vi "SP Perform Filter Ripple Limit Testing.vi"(0 "Filter Limit":T12={"Limit #"=1, "Parameter"={"Stimulus Port"=1, "Response Port"=2}, "Format"=enum."Lin Mag", "Filter Type"=enum."Bandpass", "Passband"={"Start/Center"=510.0, "Stop/Span"=610.0, "Units"=enum."MHz", "Freq Format"=enum."Start/Stop", "Bandwidth Attn"=3.0, "Passband Limit"=FALSE}, "Ripple"={"Ripple Limit"=TRUE, "Window On"=TRUE, "Ripple"=0.1, "Window"=10.0, "Units"=enum."MHz"}, "Attenuation Points"=[], "Skirt Points"=[]} {"Parameter"."Stimulus Port" min=1 step=1; "Parameter"."Response Port" min=1 step=1; "Passband"."Bandwidth Attn" format="%.3g"; "Passband"."Stop/Span" format="%.3g"; "Passband"."Start/Center" format="%.3g"}, 5 "Data":T11={"F0"=500.0, "dF"=1.0, "Formatted Values"=[-6.0, -6.0, -6.0, -6.0, -6.0, -6.0, -5.0, -4.0, -3.0, -2.0, -1.0017226002993769, -0.8636286738753696, -1.012432061728755, -0.8135188671805874, -1.084383696215112, -1.192695586219516, -0.8228939725524264, -1.1588169801015764, -1.0069715761898415, -0.8118111488159718, -0.9516999033989667, -1.0842662636672022, -1.0261931083967077, -0.816874162233468, -0.8335770068326294, -1.1794529347576463, -1.1032959879886735, -1.197742447623333, -0.9631229100196212, -0.9908453124177325, -0.9835470980893588, -1.10217991844936, -0.8956607286257672, -0.8794782872077156, -0.9013683651609963, -1.0772188731817596, -0.992723355191172, -0.9536275499498994, -0.9874327685983141, -0.921963653527827, -0.8848787728556787, -1.1874980208218, -0.996957511881206, -0.9972503730309241, -0.8866139538542095, -1.07344181331393, -0.881559772443858, -1.0112449407130875, -0.9865384477979471, -0.9901446738263366, -1.1718630063784758, -0.9951725256878827, -0.931778781153855, -0.9846289731021831, -0.851763264124267, -0.9086965469391421, -0.8349429101974368, -0.8383742350256687, -1.106571816484691, -0.9554005266395742, -0.9376822403043366, -1.131287512516927, -1.0382288806403288, -0.917054052988136, -0.9489467877812984, -0.9264227759143271, -1.0918690925892351, -1.1668737446636852, -1.0021735712381068, -1.1541225361979714, -1.1931131329605709, -0.8730502330378824, -0.850411285659811, -1.137775166801135, -1.1870586525662095, -1.0926571181161528, -1.118993526927924, -1.1211410787283602, -0.8920697041785735, -0.888430731015914, -1.0656600076605476, -1.1666787859795846, -1.0713340188424678, -0.8625910088884297, -1.1434360227216422, -0.9217710376784376, -1.1218396445954617, -0.9558195687190933, -1.1773692443654946, -1.0827782751424972, -1.1567791336122029, -0.8684407402614696, -0.8177845157195978, -0.9040657051180614, -0.9313557288389804, -1.0236831450620423, -1.050426714979035, -0.8344777069605718, -0.8274082929927138, -1.1990080831766776, -1.0947798998491134, -1.1963114865246718, -1.0016247375583676, -1.0877110100652403, -1.1556028882288836, -1.1918380581525247, -0.9751292214691399, -0.8884133044813358, -1.0347444321214612, -0.9445125246491541, -2.0, -3.0, -4.0, -5.0, -6.0, -6.0, -6.0, -6.0, -6.0, -6.0]}, 9 "Generate Plot Output? (f)":bool, 11 "error in (no error)":errorcluster, 12 "Limit Results In":T2={"Limit #"=0, "Parameter"={"Stimulus Port"=1, "Response Port"=0}, "Bandwidth Pass?"={"Pass?"=FALSE, "Bandwidth"=0.0, "Limit"=0.0, "Units"=enum."Hz"}, "Ripple Pass?"={"Pass?"=FALSE, "Ripple"=0.0, "Limit"=0.0, "Format"=enum."Log Mag"}, "Attenuation Results"=[], "Skirt Results"=[], "Pass?"=FALSE} {"Parameter"."Stimulus Port" min=1 step=1; "Parameter"."Response Port" min=1 step=1}, 13 "Format":T1 caption="Display Format" items=["Log Mag", "Phase", "Expanded Phase", "Delay", "Smith", "Polar", "Lin Mag", "SWR", "Loss", "Real", "Imaginary"]) -> (1 "Upper Limits":cluster{"x values":dbl[], "y values":dbl[]}[](array[cluster]), 3 "Lower Limits":cluster{"x values":dbl[], "y values":dbl[]}[](array[cluster]), 4 "Limits Pass/Fail":cluster{"Upper Pass?":bool, "Lower Pass?":bool}, 6 "Upper and Lower Limits":T10, 10 "Failures":cluster{"x values":dbl[], "y values":dbl[]}[](array[cluster]), 14 "Limit Results Out":T2={"Limit #"=0, "Parameter"={"Stimulus Port"=1, "Response Port"=0}, "Bandwidth Pass?"={"Pass?"=FALSE, "Bandwidth"=0.0, "Limit"=0.0, "Units"=enum."Hz"}, "Ripple Pass?"={"Pass?"=FALSE, "Ripple"=0.0, "Limit"=0.0, "Format"=enum."Log Mag"}, "Attenuation Results"=[], "Skirt Results"=[], "Pass?"=FALSE} {"Parameter"."Stimulus Port" min=1 step=1; "Parameter"."Response Port" min=1 step=1}, 15 "error out":errorcluster)   [LabVIEW 2011]
uses:
  TypeDefs/SP Filter.ctl
  TypeDefs/SP Parameter.ctl
  TypeDefs/SP Format.ctl
  TypeDefs/SP Filter Type.ctl
  TypeDefs/SP Filter Passband.ctl
  TypeDefs/SP Frequency Units.ctl
  TypeDefs/SP Frequency Format.ctl
  TypeDefs/SP Filter Ripple.ctl
  TypeDefs/SP Attenuation Point.ctl
  TypeDefs/SP Attenuation Type.ctl
  TypeDefs/SP Skirt Rejection Point.ctl
  TypeDefs/SP Relative Loss.ctl
  TypeDefs/SP Limit Results.ctl
  TypeDefs/SP Bandwidth Limit Results.ctl
  TypeDefs/SP Ripple Limit Results.ctl
  TypeDefs/SP Attenuation Limit Results.ctl
  TypeDefs/SP Skirt Limit Results.ctl
  TypeDefs/SP Display Format.ctl
panel:
  out "Plot Output":cluster{"x values":dbl[], "y values":dbl[]}[](graph)
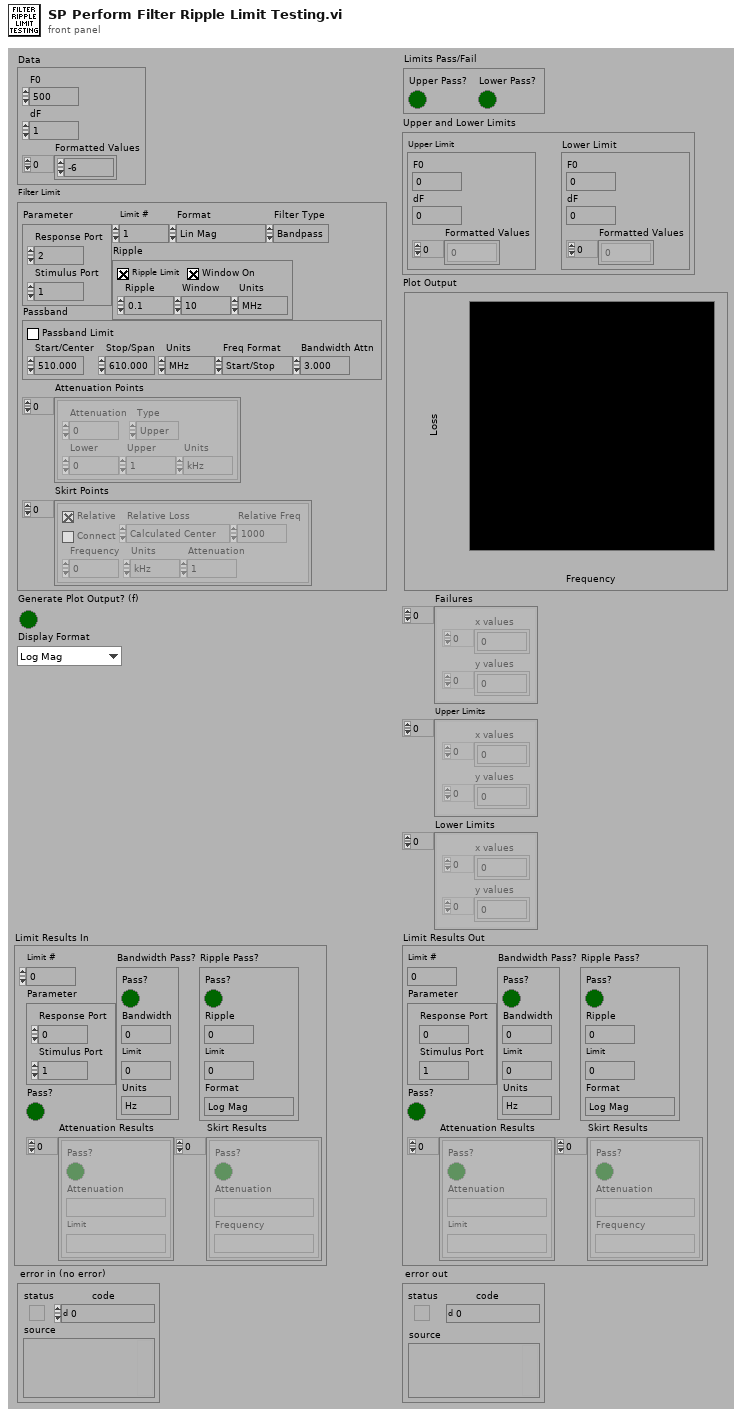
[diagram p1: front panel]
types:
  T1 = typedef "SP Display Format.ctl" = i32
  T2 = typedef "SP Limit Results.ctl" = cluster{"Limit #":i8, "Parameter":T3, "Bandwidth Pass?":T4, "Ripple Pass?":T6, "Attenuation Results":T8[], "Skirt Results":T9[], "Pass?":bool}
  T3 = typedef "SP Parameter.ctl" = cluster{"Stimulus Port":i8, "Response Port":i8}
  T4 = typedef "SP Bandwidth Limit Results.ctl" = cluster{"Pass?":bool, "Bandwidth":dbl, "Limit":dbl, "Units":T5}
  T5 = typedef "SP Frequency Units.ctl" = enum16{"Hz", "kHz", "MHz", "GHz", "Points"}
  T6 = typedef "SP Ripple Limit Results.ctl" = cluster{"Pass?":bool, "Ripple":dbl, "Limit":dbl, "Format":T7}
  T7 = typedef "SP Format.ctl" = enum16{"Log Mag", "Lin Mag", "SWR", "Phase", "Expanded Phase", "Delay", "Insertion Loss", "Isolation", "Return Loss"}
  T8 = typedef "SP Attenuation Limit Results.ctl" = cluster{"Pass?":bool, "Attenuation":string, "Limit":string}
  T9 = typedef "SP Skirt Limit Results.ctl" = cluster{"Pass?":bool, "Attenuation":string, "Frequency":string}
  T10 = cluster{"Upper Limit":cluster{"F0":dbl, "dF":dbl, "Formatted Values":dbl[]}, "Lower Limit":cluster{"F0":dbl, "dF":dbl, "Formatted Values":dbl[]}}
  T11 = cluster{"F0":dbl, "dF":dbl, "Formatted Values":dbl[]}
  T12 = typedef "SP Filter.ctl" = cluster{"Limit #":i8, "Parameter":T3, "Format":T7, "Filter Type":T13, "Passband":T14, "Ripple":T16, "Attenuation Points":T17[], "Skirt Points":T19[]}
  T13 = typedef "SP Filter Type.ctl" = enum16{"Lowpass", "Highpass", "Bandpass", "Bandstop"}
  T14 = typedef "SP Filter Passband.ctl" = cluster{"Start/Center":dbl, "Stop/Span":dbl, "Units":T5, "Freq Format":T15, "Bandwidth Attn":dbl, "Passband Limit":bool}
  T15 = typedef "SP Frequency Format.ctl" = enum16{"Start/Stop", "Center/Span"}
  T16 = typedef "SP Filter Ripple.ctl" = cluster{"Ripple Limit":bool, "Window On":bool, "Ripple":dbl, "Window":dbl, "Units":T5}
  T17 = typedef "SP Attenuation Point.ctl" = cluster{"Attenuation":dbl, "Type":T18, "Lower":dbl, "Upper":dbl, "Units":T5}
  T18 = typedef "SP Attenuation Type.ctl" = enum16{"Center", "Lower", "Upper"}
  T19 = typedef "SP Skirt Rejection Point.ctl" = cluster{"Relative":bool, "Connect":bool, "Frequency":dbl, "Units":T5, "Attenuation":dbl, "Relative Loss":T20, "Relative Freq":dbl}
  T20 = typedef "SP Relative Loss.ctl" = enum16{"Calculated Center", "Passband Minimum", "Passband Maximum", "Passband Average", "Frequency"}
  T21 = cluster{"x0":dbl, "dx":dbl, "Stored Values":dbl[]}
  T22 = cluster{cluster{"x0":dbl, "dx":dbl, "Stored Values":dbl[]}, cluster{"x0":dbl, "dx":dbl, "Stored Values":dbl[]}}
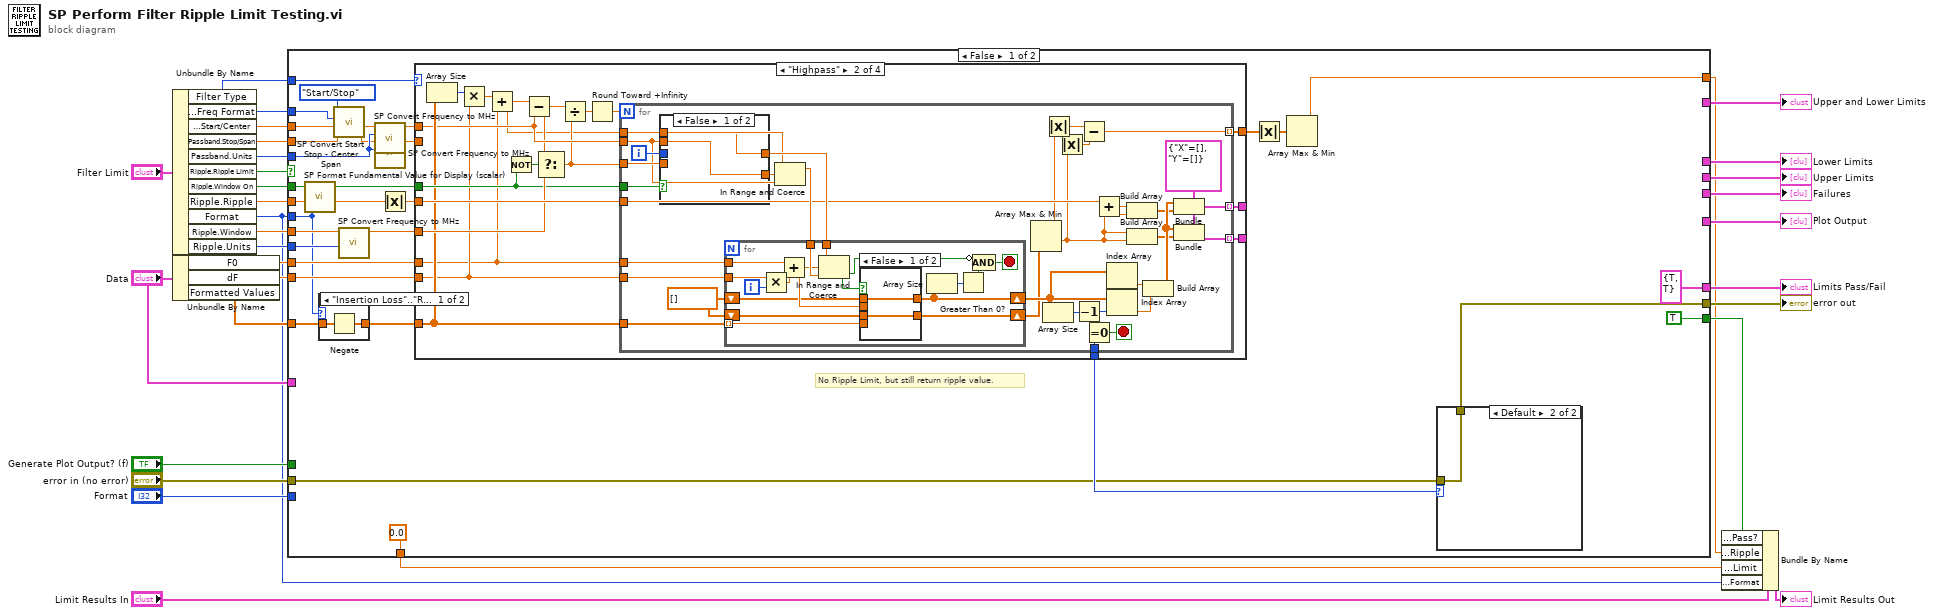
[diagram p0: block diagram]
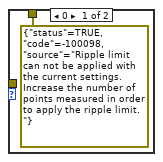
[diagram p3: hidden frame]
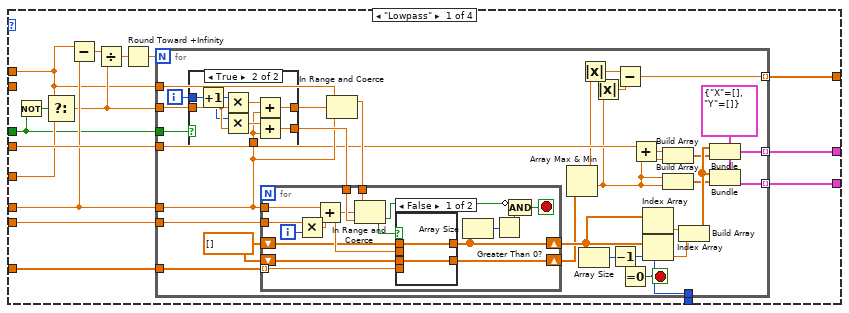
[diagram p4: hidden frame]
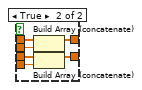
[diagram p6: hidden frame]
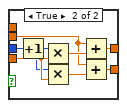
[diagram p7: hidden frame]
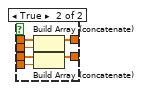
[diagram p8: hidden frame]
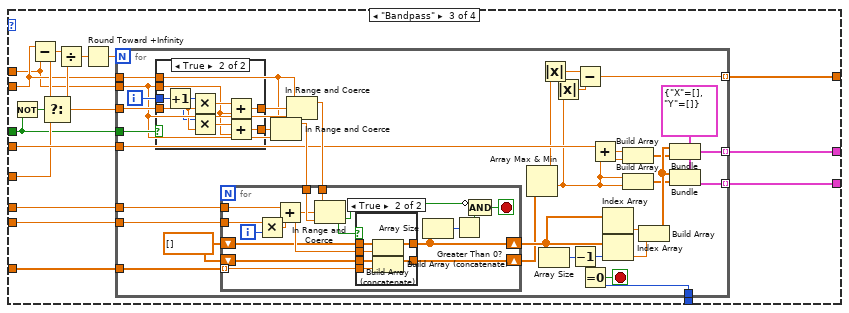
[diagram p9: hidden frame]
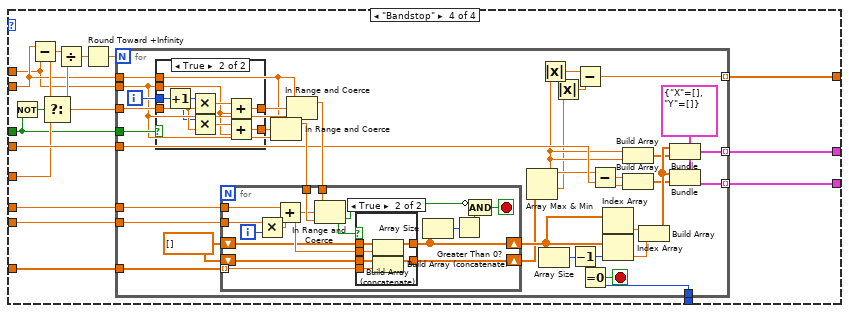
[diagram p12: hidden frame]
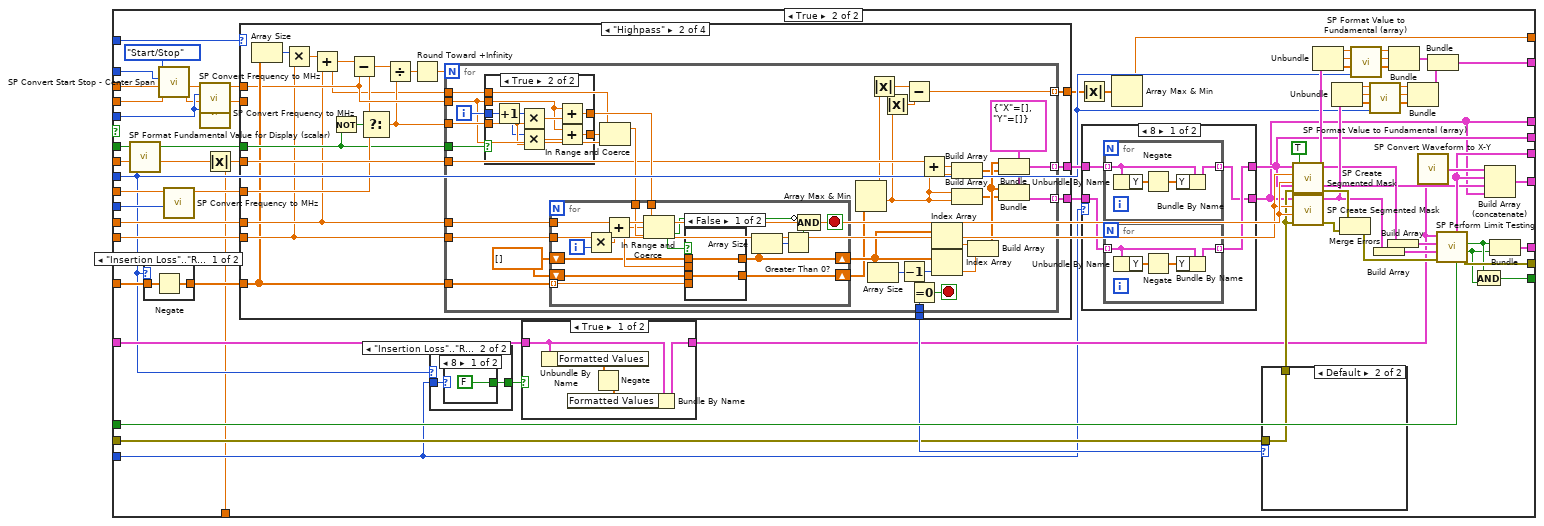
[diagram p15: hidden frame]
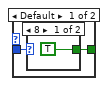
[diagram p17: hidden frame]
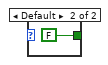
[diagram p18: hidden frame]
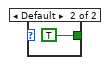
[diagram p19: hidden frame]
diagram:
  n1 = Unbundle By Name("Filter Limit") -> ("Filter Type"=w16:T13, "Passband.Freq Format"=w15:T15, "Passband.Start/Center"=w30:dbl, "Passband.Stop/Span"=w29:dbl, "Passband.Units"=w28:T5, "Ripple.Ripple Limit"=w25:bool, "Ripple.Window On"=w24:bool, "Ripple.Ripple"=w23:dbl, "Format"=w1:T7, "Ripple.Window"=w22:dbl, "Ripple.Units"=w21:T5)
  n2 = Unbundle By Name("Data") -> ("F0"=w27:dbl, "dF"=w26:dbl, "Formatted Values"=w20:dbl[])
  n3 = case shown="False" w25 {
    tunnel: w16 -> [w62 w465]
    tunnel: w30 -> [w52 w450]
    tunnel: w29 -> [w51 w449]
    tunnel: w28 -> [w61 w464]
    tunnel: w27 -> [w54 w452]
    tunnel: w26 -> [w53 w451]
    tunnel: w20 -> [w42 w418]
    tunnel: w24 -> [w55 w456]
    tunnel: w23 -> [w44 w420]
    tunnel: w22 -> [w58 w461]
    tunnel: w21 -> [w57 w460]
    tunnel: w1 -> [w40 w407]
    tunnel: "Data" -> [_ w409]
    tunnel: "Generate Plot Output? (f)" -> [_ w426]
    tunnel: [cluster{"Upper Pass?":bool, "Lower Pass?":bool} {"Upper Pass?"=TRUE, "Lower Pass?"=TRUE} w437] -> w9
    tunnel: [_ w442] -> w6
    tunnel: "error in (no error)" -> [w45 w424]
    tunnel: [w33 w458] -> w17
    tunnel: w15 -> [w47 w445]
    tunnel: [_ w412] -> w14
    tunnel: [_ w414] -> w13
    tunnel: [_ w440] -> w12
    tunnel: [TRUE w436] -> w4
    tunnel: [_ w427] -> w8
    tunnel: "Format" -> [_ w406]
    tunnel: [w37 w403] -> w3
    tunnel: [0.0 w402] -> w2
    frame False {
      # "No Ripple Limit, but still return ripple value."
      n4 = call "SP Format Fundamental Value for Display (scalar).vi"("Format"=w40, "Stored Value (0, linear)"=w44) -> ("Display Value"=w43:dbl)  [unwired: 5 out]
      n5 = case shown="\"Insertion Loss\"..\"Return Loss\"" w40 {
        tunnel: w42 -> [w64 w65]
        tunnel: [w63 w65] -> w41
        frame "Insertion Loss".."Return Loss" {
          n6 = Negate(x=w64) -> (-x=w63:dbl[])
        }
        frame Default {
        }
      }
      n7 = call "SP Convert Start Stop - Center Span.vi"("Stop/Span In"=w51, "Start/Center In"=w52, "Freq Format From"=w47, "Freq Format To"=SP_Frequency_Format."Start/Stop") -> ("Stop/Span Out"=w50:dbl, "Start/Center Out"=w49:dbl)  [unwired: 6 out]
      n8 = call "SP Convert Frequency to MHz.vi"("Units"=w57, "Frequency"=w58) -> ("Converted Frequency"=w56:dbl)  [unwired: 1 in, 8 out]
      n9 = call "SP Convert Frequency to MHz.vi"("Units"=w61, "Frequency"=w49) -> ("Converted Frequency"=w59:dbl)  [unwired: 1 in, 8 out]
      n10 = call "SP Convert Frequency to MHz.vi"("Units"=w61, "Frequency"=w50) -> ("Converted Frequency"=w60:dbl)  [unwired: 1 in, 8 out]
      n11 = Absolute Value(x=w43) -> (abs(x)=w36:dbl)
      n12 = case shown="\"Highpass\"" w62 {
        tunnel: w54 -> [w78 w153 w241 w325]
        tunnel: w53 -> [w82 w155 w242 w326]
        tunnel: w41 -> [w83 w159 w243 w327]
        tunnel: w60 -> [_ _ w238 w322]
        tunnel: w59 -> [w72 w158 w237 w321]
        tunnel: w56 -> [w79 w165 w248 w332]
        tunnel: [w71 w161 w245 w329] -> _
        tunnel: [w70 w160 w244 w328] -> _
        tunnel: w36 -> [w81 w167 w250 w334]
        tunnel: w55 -> [w73 w162 w246 w330]
        tunnel: [w69 w150 w235 w319] -> w46
        tunnel: [w68 w149 w234 w318] -> w38
        frame "Lowpass" {
          n13 = Not(x=w73) -> (.not. x?=w80:bool)
          n14 = Select(t=w72, s=w80, f=w79) -> (s? t:f=w76:dbl)
          n15 = Subtract(x=w72, y=w78) -> (x-y=w77:dbl)
          n16 = Divide(x=w77, y=w76) -> (x/y=w75:dbl)
          n17 = Round Toward +Infinity(x=w75) -> (ceil(x): smallest int >= x=w74:dbl)
          n18 = for {
            N: w74 -> [_]
            tunnel: w83 -> [w114]
            tunnel: [w106] -> w71 mode=indexing
            tunnel: [w105] -> w70 mode=indexing
            tunnel: w78 -> [w94]
            tunnel: w82 -> [w104]
            tunnel: w81 -> [w92]
            tunnel: w76 -> [w103]
            tunnel: w73 -> [w102]
            tunnel: w72 -> [w97]
            tunnel: [w89] -> w69
            tunnel: [w86] -> w68 mode=indexing
            i -> [w101]
            stop <- w90 stop-if-true
            w99 = dbl[] []
            w110 = cluster{"X":dbl[], "Y":dbl[]} {"X"=[], "Y"=[]} ("Cluster")
            n19 = case shown="True" w102 {
              tunnel: w94 -> [w116 w118]
              tunnel: [w115 w122] -> w96
              tunnel: w103 -> [w115 w121]
              tunnel: w101 -> [_ w120]
              tunnel: [w116 w117] -> w100
              frame False {
              }
              frame True {
                n20 = Increment(x=w120) -> (x+1=w124:i32)
                n21 = Multiply(x=w124, y=w121) -> (x*y=w123:dbl)
                n22 = Multiply(x=w120, y=w121) -> (x*y=w119:dbl)
                n23 = Add(x=w123, y=w118) -> (x+y=w122:dbl)
                n24 = Add(x=w119, y=w118) -> (x+y=w117:dbl)
              }
            }
            n25 = In Range and Coerce(upper limit=w97, x=w96, lower limit=w94) -> (coerced(x)=w95:dbl)  [unwired: 1 out]
            n26 = for {
              tunnel: w114 -> [w134] mode=indexing
              tunnel: w104 -> [w139]
              tunnel: w94 -> [w138]
              tunnel: w95 -> [w136]
              tunnel: w100 -> [w135]
              shift-right: [w132] -> w93
              shift-left: w99 -> [w133]
              shift-right: [w129] -> w98
              shift-left: w99 -> [w130]
              i -> [w140]
              stop <- w126 stop-if-true
              n27 = Multiply(x=w139, y=w140) -> (x*y=w137:dbl)
              n28 = Add(x=w138, y=w137) -> (x+y=w131:dbl)
              n29 = In Range and Coerce(upper limit=w136, x=w131, lower limit=w135) -> (In Range?=w127:bool)  [unwired: 1 out]
              n30 = case shown="False" w127 {
                tunnel: w134 -> [_ w148]
                tunnel: w133 -> [w142 w147]
                tunnel: [w142 w146] -> w132
                tunnel: w131 -> [_ w145]
                tunnel: w130 -> [w141 w144]
                tunnel: [w141 w143] -> w129
                frame False {
                }
                frame True {
                  n31 = Build Array (concatenate)(w144, w145) -> (w143:dbl[])
                  n32 = Build Array (concatenate)(w147, w148) -> (w146:dbl[])
                }
              }
              n33 = Array Size(array=w129) -> (size(s)=w128:i32)
              n34 = Greater Than 0?(x=w128) -> (x > 0?=w125:bool)
              n35 = Compound Arithmetic op=AND(invert w127, w125) -> (w126:bool)
            }
            n36 = Array Max & Min(array=w93) -> (max value=w84:dbl, min value=w85:dbl)  [unwired: 2 out]
            n37 = Array Size(array=w98) -> (size(s)=w113:i32)
            n38 = Absolute Value(x=w84) -> (abs(x)=w88:dbl)
            n39 = Absolute Value(x=w85) -> (abs(x)=w87:dbl)
            n40 = Decrement(x=w113) -> (x-1=w89:i32)
            n41 = Subtract(x=w88, y=w87) -> (x-y=w86:dbl)
            n42 = Equal To 0?(x=w89) -> (x = 0?=w90:bool)
            n43 = Add(x=w92, y=w85) -> (x+y=w91:dbl)
            n44 = Index Array(array=w98) -> (element=w112:dbl)  [unwired: 1 in]
            n45 = Index Array(array=w98, index=w89) -> (element=w111:dbl)
            n46 = Build Array(w91, w91) -> (w107:dbl[])
            n47 = Build Array(w85, w85) -> (w108:dbl[])
            n48 = Build Array(w112, w111) -> (w109:dbl[])
            n49 = Bundle(cluster=w110, "X"=w109, "Y"=w107) -> (w106:cluster{"X":dbl[], "Y":dbl[]})
            n50 = Bundle(cluster=w110, "X"=w109, "Y"=w108) -> (w105:cluster{"X":dbl[], "Y":dbl[]})
          }
        }
        frame "Highpass" {
          n51 = Array Size(array=w159) -> (size(s)=w156:i32)
          n52 = Multiply(x=w156, y=w155) -> (x*y=w154:dbl)
          n53 = Add(x=w154, y=w153) -> (x+y=w151:dbl)
          n54 = Not(x=w162) -> (.not. x?=w166:bool)
          n55 = Subtract(x=w151, y=w158) -> (x-y=w157:dbl)
          n56 = Select(t=w157, s=w166, f=w165) -> (s? t:f=w152:dbl)
          n57 = Divide(x=w157, y=w152) -> (x/y=w164:dbl)
          n58 = Round Toward +Infinity(x=w164) -> (ceil(x): smallest int >= x=w163:dbl)
          n59 = for {
            N: w163 -> [_]
            tunnel: w159 -> [w199]
            tunnel: [w192] -> w161 mode=indexing
            tunnel: [w191] -> w160 mode=indexing
            tunnel: w153 -> [w184]
            tunnel: w155 -> [w190]
            tunnel: w167 -> [w177]
            tunnel: w152 -> [w189]
            tunnel: w162 -> [w188]
            tunnel: w158 -> [w180]
            tunnel: w151 -> [w179]
            tunnel: [w173] -> w150
            tunnel: [w170] -> w149 mode=indexing
            i -> [w187]
            stop <- w174 stop-if-true
            w186 = dbl[] []
            w196 = cluster{"X":dbl[], "Y":dbl[]} {"X"=[], "Y"=[]} ("Cluster")
            n60 = case shown="False" w188 {
              tunnel: [w200 w207] -> w183
              tunnel: w189 -> [_ w206]
              tunnel: w187 -> [_ w205]
              tunnel: [w201 w203] -> w182
              tunnel: w180 -> [w201 w202]
              tunnel: w179 -> [w200 _]
              frame False {
              }
              frame True {
                n61 = Increment(x=w205) -> (x+1=w209:i32)
                n62 = Multiply(x=w209, y=w206) -> (x*y=w208:dbl)
                n63 = Multiply(x=w205, y=w206) -> (x*y=w204:dbl)
                n64 = Add(x=w202, y=w208) -> (x+y=w207:dbl)
                n65 = Add(x=w202, y=w204) -> (x+y=w203:dbl)
              }
            }
            n66 = In Range and Coerce(upper limit=w179, x=w182, lower limit=w180) -> (coerced(x)=w181:dbl)  [unwired: 1 out]
            n67 = for {
              tunnel: w199 -> [w219] mode=indexing
              tunnel: w190 -> [w224]
              tunnel: w184 -> [w223]
              tunnel: w183 -> [w221]
              tunnel: w181 -> [w220]
              shift-right: [w217] -> w178
              shift-left: w186 -> [w218]
              shift-right: [w214] -> w185
              shift-left: w186 -> [w215]
              i -> [w225]
              stop <- w211 stop-if-true
              n68 = Multiply(x=w224, y=w225) -> (x*y=w222:dbl)
              n69 = Add(x=w223, y=w222) -> (x+y=w216:dbl)
              n70 = In Range and Coerce(upper limit=w221, x=w216, lower limit=w220) -> (In Range?=w212:bool)  [unwired: 1 out]
              n71 = case shown="False" w212 {
                tunnel: w219 -> [_ w233]
                tunnel: w218 -> [w227 w232]
                tunnel: [w227 w231] -> w217
                tunnel: w216 -> [_ w230]
                tunnel: w215 -> [w226 w229]
                tunnel: [w226 w228] -> w214
                frame False {
                }
                frame True {
                  n72 = Build Array (concatenate)(w229, w230) -> (w228:dbl[])
                  n73 = Build Array (concatenate)(w232, w233) -> (w231:dbl[])
                }
              }
              n74 = Array Size(array=w214) -> (size(s)=w213:i32)
              n75 = Greater Than 0?(x=w213) -> (x > 0?=w210:bool)
              n76 = Compound Arithmetic op=AND(invert w212, w210) -> (w211:bool)
            }
            n77 = Array Max & Min(array=w178) -> (max value=w168:dbl, min value=w169:dbl)  [unwired: 2 out]
            n78 = Array Size(array=w185) -> (size(s)=w175:i32)
            n79 = Absolute Value(x=w168) -> (abs(x)=w172:dbl)
            n80 = Absolute Value(x=w169) -> (abs(x)=w171:dbl)
            n81 = Decrement(x=w175) -> (x-1=w173:i32)
            n82 = Subtract(x=w172, y=w171) -> (x-y=w170:dbl)
            n83 = Equal To 0?(x=w173) -> (x = 0?=w174:bool)
            n84 = Add(x=w177, y=w169) -> (x+y=w176:dbl)
            n85 = Index Array(array=w185) -> (element=w198:dbl)  [unwired: 1 in]
            n86 = Index Array(array=w185, index=w173) -> (element=w197:dbl)
            n87 = Build Array(w176, w176) -> (w193:dbl[])
            n88 = Build Array(w169, w169) -> (w194:dbl[])
            n89 = Build Array(w198, w197) -> (w195:dbl[])
            n90 = Bundle(cluster=w196, "X"=w195, "Y"=w193) -> (w192:cluster{"X":dbl[], "Y":dbl[]})
            n91 = Bundle(cluster=w196, "X"=w195, "Y"=w194) -> (w191:cluster{"X":dbl[], "Y":dbl[]})
          }
        }
        frame "Bandpass" {
          n92 = Not(x=w246) -> (.not. x?=w249:bool)
          n93 = Subtract(x=w238, y=w237) -> (x-y=w239:dbl)
          n94 = Select(t=w239, s=w249, f=w248) -> (s? t:f=w240:dbl)
          n95 = Divide(x=w239, y=w240) -> (x/y=w247:dbl)
          n96 = Round Toward +Infinity(x=w247) -> (ceil(x): smallest int >= x=w236:dbl)
          n97 = for {
            N: w236 -> [_]
            tunnel: w243 -> [w283]
            tunnel: [w276] -> w245 mode=indexing
            tunnel: [w275] -> w244 mode=indexing
            tunnel: w241 -> [w268]
            tunnel: w242 -> [w274]
            tunnel: w250 -> [w259]
            tunnel: w240 -> [w273]
            tunnel: w246 -> [w272]
            tunnel: w237 -> [w263]
            tunnel: w238 -> [w262]
            tunnel: [w256] -> w235
            tunnel: [w255] -> w234 mode=indexing
            i -> [w271]
            stop <- w257 stop-if-true
            w270 = dbl[] []
            w280 = cluster{"X":dbl[], "Y":dbl[]} {"X"=[], "Y"=[]} ("Cluster")
            n98 = case shown="True" w272 {
              tunnel: [w284 w291] -> w265
              tunnel: w273 -> [_ w290]
              tunnel: w271 -> [_ w289]
              tunnel: [w285 w287] -> w267
              tunnel: w263 -> [w285 w286]
              tunnel: w262 -> [w284 _]
              frame False {
              }
              frame True {
                n99 = Increment(x=w289) -> (x+1=w293:i32)
                n100 = Multiply(x=w293, y=w290) -> (x*y=w292:dbl)
                n101 = Multiply(x=w289, y=w290) -> (x*y=w288:dbl)
                n102 = Add(x=w292, y=w286) -> (x+y=w291:dbl)
                n103 = Add(x=w288, y=w286) -> (x+y=w287:dbl)
              }
            }
            n104 = In Range and Coerce(upper limit=w262, x=w267, lower limit=w263) -> (coerced(x)=w266:dbl)  [unwired: 1 out]
            n105 = In Range and Coerce(upper limit=w262, x=w265, lower limit=w263) -> (coerced(x)=w264:dbl)  [unwired: 1 out]
            n106 = for {
              tunnel: w283 -> [w303] mode=indexing
              tunnel: w274 -> [w308]
              tunnel: w268 -> [w307]
              tunnel: w264 -> [w305]
              tunnel: w266 -> [w304]
              shift-right: [w301] -> w261
              shift-left: w270 -> [w302]
              shift-right: [w298] -> w269
              shift-left: w270 -> [w299]
              i -> [w309]
              stop <- w295 stop-if-true
              n107 = Multiply(x=w308, y=w309) -> (x*y=w306:dbl)
              n108 = Add(x=w307, y=w306) -> (x+y=w300:dbl)
              n109 = In Range and Coerce(upper limit=w305, x=w300, lower limit=w304) -> (In Range?=w296:bool)  [unwired: 1 out]
              n110 = case shown="True" w296 {
                tunnel: w303 -> [_ w317]
                tunnel: w302 -> [w311 w316]
                tunnel: [w311 w315] -> w301
                tunnel: w300 -> [_ w314]
                tunnel: w299 -> [w310 w313]
                tunnel: [w310 w312] -> w298
                frame False {
                }
                frame True {
                  n111 = Build Array (concatenate)(w313, w314) -> (w312:dbl[])
                  n112 = Build Array (concatenate)(w316, w317) -> (w315:dbl[])
                }
              }
              n113 = Array Size(array=w298) -> (size(s)=w297:i32)
              n114 = Greater Than 0?(x=w297) -> (x > 0?=w294:bool)
              n115 = Compound Arithmetic op=AND(invert w296, w294) -> (w295:bool)
            }
            n116 = Array Max & Min(array=w261) -> (max value=w254:dbl, min value=w252:dbl)  [unwired: 2 out]
            n117 = Array Size(array=w269) -> (size(s)=w258:i32)
            n118 = Absolute Value(x=w254) -> (abs(x)=w253:dbl)
            n119 = Absolute Value(x=w252) -> (abs(x)=w251:dbl)
            n120 = Decrement(x=w258) -> (x-1=w256:i32)
            n121 = Subtract(x=w253, y=w251) -> (x-y=w255:dbl)
            n122 = Equal To 0?(x=w256) -> (x = 0?=w257:bool)
            n123 = Add(x=w259, y=w252) -> (x+y=w260:dbl)
            n124 = Index Array(array=w269) -> (element=w282:dbl)  [unwired: 1 in]
            n125 = Index Array(array=w269, index=w256) -> (element=w281:dbl)
            n126 = Build Array(w260, w260) -> (w277:dbl[])
            n127 = Build Array(w252, w252) -> (w278:dbl[])
            n128 = Build Array(w282, w281) -> (w279:dbl[])
            n129 = Bundle(cluster=w280, "X"=w279, "Y"=w277) -> (w276:cluster{"X":dbl[], "Y":dbl[]})
            n130 = Bundle(cluster=w280, "X"=w279, "Y"=w278) -> (w275:cluster{"X":dbl[], "Y":dbl[]})
          }
        }
        frame "Bandstop" {
          n131 = Not(x=w330) -> (.not. x?=w333:bool)
          n132 = Subtract(x=w322, y=w321) -> (x-y=w323:dbl)
          n133 = Select(t=w323, s=w333, f=w332) -> (s? t:f=w324:dbl)
          n134 = Divide(x=w323, y=w324) -> (x/y=w331:dbl)
          n135 = Round Toward +Infinity(x=w331) -> (ceil(x): smallest int >= x=w320:dbl)
          n136 = for {
            N: w320 -> [_]
            tunnel: w327 -> [w367]
            tunnel: [w358] -> w329 mode=indexing
            tunnel: [w357] -> w328 mode=indexing
            tunnel: w325 -> [w350]
            tunnel: w326 -> [w356]
            tunnel: w334 -> [w342]
            tunnel: w324 -> [w355]
            tunnel: w330 -> [w354]
            tunnel: w321 -> [w345]
            tunnel: w322 -> [w344]
            tunnel: [w340] -> w319
            tunnel: [w335] -> w318 mode=indexing
            i -> [w353]
            stop <- w341 stop-if-true
            w352 = dbl[] []
            w362 = cluster{"X":dbl[], "Y":dbl[]} {"X"=[], "Y"=[]} ("Cluster")
            n137 = case shown="True" w354 {
              tunnel: [w368 w375] -> w347
              tunnel: w355 -> [_ w374]
              tunnel: w353 -> [_ w373]
              tunnel: [w369 w371] -> w349
              tunnel: w345 -> [w369 w370]
              tunnel: w344 -> [w368 _]
              frame False {
              }
              frame True {
                n138 = Increment(x=w373) -> (x+1=w377:i32)
                n139 = Multiply(x=w377, y=w374) -> (x*y=w376:dbl)
                n140 = Multiply(x=w373, y=w374) -> (x*y=w372:dbl)
                n141 = Add(x=w376, y=w370) -> (x+y=w375:dbl)
                n142 = Add(x=w372, y=w370) -> (x+y=w371:dbl)
              }
            }
            n143 = In Range and Coerce(upper limit=w344, x=w349, lower limit=w345) -> (coerced(x)=w348:dbl)  [unwired: 1 out]
            n144 = In Range and Coerce(upper limit=w344, x=w347, lower limit=w345) -> (coerced(x)=w346:dbl)  [unwired: 1 out]
            n145 = for {
              tunnel: w367 -> [w387] mode=indexing
              tunnel: w356 -> [w392]
              tunnel: w350 -> [w391]
              tunnel: w346 -> [w389]
              tunnel: w348 -> [w388]
              shift-right: [w385] -> w343
              shift-left: w352 -> [w386]
              shift-right: [w382] -> w351
              shift-left: w352 -> [w383]
              i -> [w393]
              stop <- w379 stop-if-true
              n146 = Multiply(x=w392, y=w393) -> (x*y=w390:dbl)
              n147 = Add(x=w391, y=w390) -> (x+y=w384:dbl)
              n148 = In Range and Coerce(upper limit=w389, x=w384, lower limit=w388) -> (In Range?=w380:bool)  [unwired: 1 out]
              n149 = case shown="True" w380 {
                tunnel: w387 -> [_ w401]
                tunnel: w386 -> [w395 w400]
                tunnel: [w395 w399] -> w385
                tunnel: w384 -> [_ w398]
                tunnel: w383 -> [w394 w397]
                tunnel: [w394 w396] -> w382
                frame False {
                }
                frame True {
                  n150 = Build Array (concatenate)(w397, w398) -> (w396:dbl[])
                  n151 = Build Array (concatenate)(w400, w401) -> (w399:dbl[])
                }
              }
              n152 = Array Size(array=w382) -> (size(s)=w381:i32)
              n153 = Greater Than 0?(x=w381) -> (x > 0?=w378:bool)
              n154 = Compound Arithmetic op=AND(invert w380, w378) -> (w379:bool)
            }
            n155 = Array Max & Min(array=w343) -> (max value=w337:dbl, min value=w336:dbl)  [unwired: 2 out]
            n156 = Array Size(array=w351) -> (size(s)=w366:i32)
            n157 = Absolute Value(x=w337) -> (abs(x)=w339:dbl)
            n158 = Absolute Value(x=w336) -> (abs(x)=w338:dbl)
            n159 = Decrement(x=w366) -> (x-1=w340:i32)
            n160 = Subtract(x=w339, y=w338) -> (x-y=w335:dbl)
            n161 = Equal To 0?(x=w340) -> (x = 0?=w341:bool)
            n162 = Subtract(x=w337, y=w342) -> (x-y=w363:dbl)
            n163 = Index Array(array=w351) -> (element=w365:dbl)  [unwired: 1 in]
            n164 = Index Array(array=w351, index=w340) -> (element=w364:dbl)
            n165 = Build Array(w337, w337) -> (w359:dbl[])
            n166 = Build Array(w363, w363) -> (w360:dbl[])
            n167 = Build Array(w365, w364) -> (w361:dbl[])
            n168 = Bundle(cluster=w362, "X"=w361, "Y"=w359) -> (w358:cluster{"X":dbl[], "Y":dbl[]})
            n169 = Bundle(cluster=w362, "X"=w361, "Y"=w360) -> (w357:cluster{"X":dbl[], "Y":dbl[]})
          }
        }
      }
      n170 = Absolute Value(x=w38) -> (abs(x)=w39:dbl[])
      n171 = Array Max & Min(array=w39) -> (max value=w37:dbl)  [unwired: 3 out]
      n172 = case shown="Default" w46 {
        tunnel: w45 -> [_ w67]
        tunnel: [errorcluster {"status"=TRUE, "code"=-100098, "source"="Ripple limit can not be applied with the current settings.  Increase the number of points measured in order to apply the ripple limit."} ("error in (no error)") w67] -> w33
        frame 0 {
        }
        frame Default {
        }
      }
    }
    frame True {
      w455 = TRUE ("Reset")
      n173 = call "SP Format Fundamental Value for Display (scalar).vi"("Format"=w407, "Stored Value (0, linear)"=w420) -> ("Display Value"=w419:dbl)  [unwired: 5 out]
      n174 = case shown="\"Insertion Loss\"..\"Return Loss\"" w407 {
        tunnel: w418 -> [w494 w495]
        tunnel: [w493 w495] -> w411
        frame "Insertion Loss".."Return Loss" {
          n175 = Negate(x=w494) -> (-x=w493:dbl[])
        }
        frame Default {
        }
      }
      n176 = call "SP Convert Start Stop - Center Span.vi"("Stop/Span In"=w449, "Start/Center In"=w450, "Freq Format From"=w445, "Freq Format To"=SP_Frequency_Format."Start/Stop") -> ("Stop/Span Out"=w448:dbl, "Start/Center Out"=w447:dbl)  [unwired: 6 out]
      n177 = call "SP Convert Frequency to MHz.vi"("Units"=w460, "Frequency"=w461) -> ("Converted Frequency"=w459:dbl)  [unwired: 1 in, 8 out]
      n178 = call "SP Convert Frequency to MHz.vi"("Units"=w464, "Frequency"=w447) -> ("Converted Frequency"=w462:dbl)  [unwired: 1 in, 8 out]
      n179 = call "SP Convert Frequency to MHz.vi"("Units"=w464, "Frequency"=w448) -> ("Converted Frequency"=w463:dbl)  [unwired: 1 in, 8 out]
      n180 = Absolute Value(x=w419) -> (abs(x)=w402:dbl)
      n181 = case shown="\"Highpass\"" w465 {
        tunnel: w452 -> [w508 w583 w671 w755]
        tunnel: w451 -> [w512 w585 w672 w756]
        tunnel: w411 -> [w513 w589 w673 w757]
        tunnel: w463 -> [_ _ w668 w752]
        tunnel: w462 -> [w502 w588 w667 w751]
        tunnel: w459 -> [w509 w595 w678 w762]
        tunnel: [w501 w591 w675 w759] -> w415
        tunnel: [w500 w590 w674 w758] -> w413
        tunnel: w402 -> [w511 w597 w680 w764]
        tunnel: w456 -> [w503 w592 w676 w760]
        tunnel: [w499 w580 w665 w749] -> w425
        tunnel: [w498 w579 w664 w748] -> w404
        frame "Lowpass" {
          n182 = Not(x=w503) -> (.not. x?=w510:bool)
          n183 = Select(t=w502, s=w510, f=w509) -> (s? t:f=w506:dbl)
          n184 = Subtract(x=w502, y=w508) -> (x-y=w507:dbl)
          n185 = Divide(x=w507, y=w506) -> (x/y=w505:dbl)
          n186 = Round Toward +Infinity(x=w505) -> (ceil(x): smallest int >= x=w504:dbl)
          n187 = for {
            N: w504 -> [_]
            tunnel: w513 -> [w544]
            tunnel: [w536] -> w501 mode=indexing
            tunnel: [w535] -> w500 mode=indexing
            tunnel: w508 -> [w524]
            tunnel: w512 -> [w534]
            tunnel: w511 -> [w522]
            tunnel: w506 -> [w533]
            tunnel: w503 -> [w532]
            tunnel: w502 -> [w527]
            tunnel: [w519] -> w499
            tunnel: [w516] -> w498 mode=indexing
            i -> [w531]
            stop <- w520 stop-if-true
            w529 = dbl[] []
            w540 = cluster{"X":dbl[], "Y":dbl[]} {"X"=[], "Y"=[]} ("Cluster")
            n188 = case shown="True" w532 {
              tunnel: w524 -> [w546 w548]
              tunnel: [w545 w552] -> w526
              tunnel: w533 -> [w545 w551]
              tunnel: w531 -> [_ w550]
              tunnel: [w546 w547] -> w530
              frame False {
              }
              frame True {
                n189 = Increment(x=w550) -> (x+1=w554:i32)
                n190 = Multiply(x=w554, y=w551) -> (x*y=w553:dbl)
                n191 = Multiply(x=w550, y=w551) -> (x*y=w549:dbl)
                n192 = Add(x=w553, y=w548) -> (x+y=w552:dbl)
                n193 = Add(x=w549, y=w548) -> (x+y=w547:dbl)
              }
            }
            n194 = In Range and Coerce(upper limit=w527, x=w526, lower limit=w524) -> (coerced(x)=w525:dbl)  [unwired: 1 out]
            n195 = for {
              tunnel: w544 -> [w564] mode=indexing
              tunnel: w534 -> [w569]
              tunnel: w524 -> [w568]
              tunnel: w525 -> [w566]
              tunnel: w530 -> [w565]
              shift-right: [w562] -> w523
              shift-left: w529 -> [w563]
              shift-right: [w559] -> w528
              shift-left: w529 -> [w560]
              i -> [w570]
              stop <- w556 stop-if-true
              n196 = Multiply(x=w569, y=w570) -> (x*y=w567:dbl)
              n197 = Add(x=w568, y=w567) -> (x+y=w561:dbl)
              n198 = In Range and Coerce(upper limit=w566, x=w561, lower limit=w565) -> (In Range?=w557:bool)  [unwired: 1 out]
              n199 = case shown="False" w557 {
                tunnel: w564 -> [_ w578]
                tunnel: w563 -> [w572 w577]
                tunnel: [w572 w576] -> w562
                tunnel: w561 -> [_ w575]
                tunnel: w560 -> [w571 w574]
                tunnel: [w571 w573] -> w559
                frame False {
                }
                frame True {
                  n200 = Build Array (concatenate)(w574, w575) -> (w573:dbl[])
                  n201 = Build Array (concatenate)(w577, w578) -> (w576:dbl[])
                }
              }
              n202 = Array Size(array=w559) -> (size(s)=w558:i32)
              n203 = Greater Than 0?(x=w558) -> (x > 0?=w555:bool)
              n204 = Compound Arithmetic op=AND(invert w557, w555) -> (w556:bool)
            }
            n205 = Array Max & Min(array=w523) -> (max value=w514:dbl, min value=w515:dbl)  [unwired: 2 out]
            n206 = Array Size(array=w528) -> (size(s)=w543:i32)
            n207 = Absolute Value(x=w514) -> (abs(x)=w518:dbl)
            n208 = Absolute Value(x=w515) -> (abs(x)=w517:dbl)
            n209 = Decrement(x=w543) -> (x-1=w519:i32)
            n210 = Subtract(x=w518, y=w517) -> (x-y=w516:dbl)
            n211 = Equal To 0?(x=w519) -> (x = 0?=w520:bool)
            n212 = Add(x=w522, y=w515) -> (x+y=w521:dbl)
            n213 = Index Array(array=w528) -> (element=w542:dbl)  [unwired: 1 in]
            n214 = Index Array(array=w528, index=w519) -> (element=w541:dbl)
            n215 = Build Array(w521, w521) -> (w537:dbl[])
            n216 = Build Array(w515, w515) -> (w538:dbl[])
            n217 = Build Array(w542, w541) -> (w539:dbl[])
            n218 = Bundle(cluster=w540, "X"=w539, "Y"=w537) -> (w536:cluster{"X":dbl[], "Y":dbl[]})
            n219 = Bundle(cluster=w540, "X"=w539, "Y"=w538) -> (w535:cluster{"X":dbl[], "Y":dbl[]})
          }
        }
        frame "Highpass" {
          n220 = Array Size(array=w589) -> (size(s)=w586:i32)
          n221 = Multiply(x=w586, y=w585) -> (x*y=w584:dbl)
          n222 = Add(x=w584, y=w583) -> (x+y=w581:dbl)
          n223 = Not(x=w592) -> (.not. x?=w596:bool)
          n224 = Subtract(x=w581, y=w588) -> (x-y=w587:dbl)
          n225 = Select(t=w587, s=w596, f=w595) -> (s? t:f=w582:dbl)
          n226 = Divide(x=w587, y=w582) -> (x/y=w594:dbl)
          n227 = Round Toward +Infinity(x=w594) -> (ceil(x): smallest int >= x=w593:dbl)
          n228 = for {
            N: w593 -> [_]
            tunnel: w589 -> [w629]
            tunnel: [w622] -> w591 mode=indexing
            tunnel: [w621] -> w590 mode=indexing
            tunnel: w583 -> [w614]
            tunnel: w585 -> [w620]
            tunnel: w597 -> [w607]
            tunnel: w582 -> [w619]
            tunnel: w592 -> [w618]
            tunnel: w588 -> [w610]
            tunnel: w581 -> [w609]
            tunnel: [w603] -> w580
            tunnel: [w600] -> w579 mode=indexing
            i -> [w617]
            stop <- w604 stop-if-true
            w616 = dbl[] []
            w626 = cluster{"X":dbl[], "Y":dbl[]} {"X"=[], "Y"=[]} ("Cluster")
            n229 = case shown="True" w618 {
              tunnel: [w630 w637] -> w613
              tunnel: w619 -> [_ w636]
              tunnel: w617 -> [_ w635]
              tunnel: [w631 w633] -> w612
              tunnel: w610 -> [w631 w632]
              tunnel: w609 -> [w630 _]
              frame False {
              }
              frame True {
                n230 = Increment(x=w635) -> (x+1=w639:i32)
                n231 = Multiply(x=w639, y=w636) -> (x*y=w638:dbl)
                n232 = Multiply(x=w635, y=w636) -> (x*y=w634:dbl)
                n233 = Add(x=w632, y=w638) -> (x+y=w637:dbl)
                n234 = Add(x=w632, y=w634) -> (x+y=w633:dbl)
              }
            }
            n235 = In Range and Coerce(upper limit=w609, x=w612, lower limit=w610) -> (coerced(x)=w611:dbl)  [unwired: 1 out]
            n236 = for {
              tunnel: w629 -> [w649] mode=indexing
              tunnel: w620 -> [w654]
              tunnel: w614 -> [w653]
              tunnel: w613 -> [w651]
              tunnel: w611 -> [w650]
              shift-right: [w647] -> w608
              shift-left: w616 -> [w648]
              shift-right: [w644] -> w615
              shift-left: w616 -> [w645]
              i -> [w655]
              stop <- w641 stop-if-true
              n237 = Multiply(x=w654, y=w655) -> (x*y=w652:dbl)
              n238 = Add(x=w653, y=w652) -> (x+y=w646:dbl)
              n239 = In Range and Coerce(upper limit=w651, x=w646, lower limit=w650) -> (In Range?=w642:bool)  [unwired: 1 out]
              n240 = case shown="False" w642 {
                tunnel: w649 -> [_ w663]
                tunnel: w648 -> [w657 w662]
                tunnel: [w657 w661] -> w647
                tunnel: w646 -> [_ w660]
                tunnel: w645 -> [w656 w659]
                tunnel: [w656 w658] -> w644
                frame False {
                }
                frame True {
                  n241 = Build Array (concatenate)(w659, w660) -> (w658:dbl[])
                  n242 = Build Array (concatenate)(w662, w663) -> (w661:dbl[])
                }
              }
              n243 = Array Size(array=w644) -> (size(s)=w643:i32)
              n244 = Greater Than 0?(x=w643) -> (x > 0?=w640:bool)
              n245 = Compound Arithmetic op=AND(invert w642, w640) -> (w641:bool)
            }
            n246 = Array Max & Min(array=w608) -> (max value=w598:dbl, min value=w599:dbl)  [unwired: 2 out]
            n247 = Array Size(array=w615) -> (size(s)=w605:i32)
            n248 = Absolute Value(x=w598) -> (abs(x)=w602:dbl)
            n249 = Absolute Value(x=w599) -> (abs(x)=w601:dbl)
            n250 = Decrement(x=w605) -> (x-1=w603:i32)
            n251 = Subtract(x=w602, y=w601) -> (x-y=w600:dbl)
            n252 = Equal To 0?(x=w603) -> (x = 0?=w604:bool)
            n253 = Add(x=w607, y=w599) -> (x+y=w606:dbl)
            n254 = Index Array(array=w615) -> (element=w628:dbl)  [unwired: 1 in]
            n255 = Index Array(array=w615, index=w603) -> (element=w627:dbl)
            n256 = Build Array(w606, w606) -> (w623:dbl[])
            n257 = Build Array(w599, w599) -> (w624:dbl[])
            n258 = Build Array(w628, w627) -> (w625:dbl[])
            n259 = Bundle(cluster=w626, "X"=w625, "Y"=w623) -> (w622:cluster{"X":dbl[], "Y":dbl[]})
            n260 = Bundle(cluster=w626, "X"=w625, "Y"=w624) -> (w621:cluster{"X":dbl[], "Y":dbl[]})
          }
        }
        frame "Bandpass" {
          n261 = Not(x=w676) -> (.not. x?=w679:bool)
          n262 = Subtract(x=w668, y=w667) -> (x-y=w669:dbl)
          n263 = Select(t=w669, s=w679, f=w678) -> (s? t:f=w670:dbl)
          n264 = Divide(x=w669, y=w670) -> (x/y=w677:dbl)
          n265 = Round Toward +Infinity(x=w677) -> (ceil(x): smallest int >= x=w666:dbl)
          n266 = for {
            N: w666 -> [_]
            tunnel: w673 -> [w713]
            tunnel: [w706] -> w675 mode=indexing
            tunnel: [w705] -> w674 mode=indexing
            tunnel: w671 -> [w698]
            tunnel: w672 -> [w704]
            tunnel: w680 -> [w689]
            tunnel: w670 -> [w703]
            tunnel: w676 -> [w702]
            tunnel: w667 -> [w693]
            tunnel: w668 -> [w692]
            tunnel: [w686] -> w665
            tunnel: [w685] -> w664 mode=indexing
            i -> [w701]
            stop <- w687 stop-if-true
            w700 = dbl[] []
            w710 = cluster{"X":dbl[], "Y":dbl[]} {"X"=[], "Y"=[]} ("Cluster")
            n267 = case shown="True" w702 {
              tunnel: [w714 w721] -> w695
              tunnel: w703 -> [_ w720]
              tunnel: w701 -> [_ w719]
              tunnel: [w715 w717] -> w697
              tunnel: w693 -> [w715 w716]
              tunnel: w692 -> [w714 _]
              frame False {
              }
              frame True {
                n268 = Increment(x=w719) -> (x+1=w723:i32)
                n269 = Multiply(x=w723, y=w720) -> (x*y=w722:dbl)
                n270 = Multiply(x=w719, y=w720) -> (x*y=w718:dbl)
                n271 = Add(x=w722, y=w716) -> (x+y=w721:dbl)
                n272 = Add(x=w718, y=w716) -> (x+y=w717:dbl)
              }
            }
            n273 = In Range and Coerce(upper limit=w692, x=w697, lower limit=w693) -> (coerced(x)=w696:dbl)  [unwired: 1 out]
            n274 = In Range and Coerce(upper limit=w692, x=w695, lower limit=w693) -> (coerced(x)=w694:dbl)  [unwired: 1 out]
            n275 = for {
              tunnel: w713 -> [w733] mode=indexing
              tunnel: w704 -> [w738]
              tunnel: w698 -> [w737]
              tunnel: w694 -> [w735]
              tunnel: w696 -> [w734]
              shift-right: [w731] -> w691
              shift-left: w700 -> [w732]
              shift-right: [w728] -> w699
              shift-left: w700 -> [w729]
              i -> [w739]
              stop <- w725 stop-if-true
              n276 = Multiply(x=w738, y=w739) -> (x*y=w736:dbl)
              n277 = Add(x=w737, y=w736) -> (x+y=w730:dbl)
              n278 = In Range and Coerce(upper limit=w735, x=w730, lower limit=w734) -> (In Range?=w726:bool)  [unwired: 1 out]
              n279 = case shown="True" w726 {
                tunnel: w733 -> [_ w747]
                tunnel: w732 -> [w741 w746]
                tunnel: [w741 w745] -> w731
                tunnel: w730 -> [_ w744]
                tunnel: w729 -> [w740 w743]
                tunnel: [w740 w742] -> w728
                frame False {
                }
                frame True {
                  n280 = Build Array (concatenate)(w743, w744) -> (w742:dbl[])
                  n281 = Build Array (concatenate)(w746, w747) -> (w745:dbl[])
                }
              }
              n282 = Array Size(array=w728) -> (size(s)=w727:i32)
              n283 = Greater Than 0?(x=w727) -> (x > 0?=w724:bool)
              n284 = Compound Arithmetic op=AND(invert w726, w724) -> (w725:bool)
            }
            n285 = Array Max & Min(array=w691) -> (max value=w684:dbl, min value=w682:dbl)  [unwired: 2 out]
            n286 = Array Size(array=w699) -> (size(s)=w688:i32)
            n287 = Absolute Value(x=w684) -> (abs(x)=w683:dbl)
            n288 = Absolute Value(x=w682) -> (abs(x)=w681:dbl)
            n289 = Decrement(x=w688) -> (x-1=w686:i32)
            n290 = Subtract(x=w683, y=w681) -> (x-y=w685:dbl)
            n291 = Equal To 0?(x=w686) -> (x = 0?=w687:bool)
            n292 = Add(x=w689, y=w682) -> (x+y=w690:dbl)
            n293 = Index Array(array=w699) -> (element=w712:dbl)  [unwired: 1 in]
            n294 = Index Array(array=w699, index=w686) -> (element=w711:dbl)
            n295 = Build Array(w690, w690) -> (w707:dbl[])
            n296 = Build Array(w682, w682) -> (w708:dbl[])
            n297 = Build Array(w712, w711) -> (w709:dbl[])
            n298 = Bundle(cluster=w710, "X"=w709, "Y"=w707) -> (w706:cluster{"X":dbl[], "Y":dbl[]})
            n299 = Bundle(cluster=w710, "X"=w709, "Y"=w708) -> (w705:cluster{"X":dbl[], "Y":dbl[]})
          }
        }
        frame "Bandstop" {
          n300 = Not(x=w760) -> (.not. x?=w763:bool)
          n301 = Subtract(x=w752, y=w751) -> (x-y=w753:dbl)
          n302 = Select(t=w753, s=w763, f=w762) -> (s? t:f=w754:dbl)
          n303 = Divide(x=w753, y=w754) -> (x/y=w761:dbl)
          n304 = Round Toward +Infinity(x=w761) -> (ceil(x): smallest int >= x=w750:dbl)
          n305 = for {
            N: w750 -> [_]
            tunnel: w757 -> [w797]
            tunnel: [w788] -> w759 mode=indexing
            tunnel: [w787] -> w758 mode=indexing
            tunnel: w755 -> [w780]
            tunnel: w756 -> [w786]
            tunnel: w764 -> [w772]
            tunnel: w754 -> [w785]
            tunnel: w760 -> [w784]
            tunnel: w751 -> [w775]
            tunnel: w752 -> [w774]
            tunnel: [w770] -> w749
            tunnel: [w765] -> w748 mode=indexing
            i -> [w783]
            stop <- w771 stop-if-true
            w782 = dbl[] []
            w792 = cluster{"X":dbl[], "Y":dbl[]} {"X"=[], "Y"=[]} ("Cluster")
            n306 = case shown="True" w784 {
              tunnel: [w798 w805] -> w777
              tunnel: w785 -> [_ w804]
              tunnel: w783 -> [_ w803]
              tunnel: [w799 w801] -> w779
              tunnel: w775 -> [w799 w800]
              tunnel: w774 -> [w798 _]
              frame False {
              }
              frame True {
                n307 = Increment(x=w803) -> (x+1=w807:i32)
                n308 = Multiply(x=w807, y=w804) -> (x*y=w806:dbl)
                n309 = Multiply(x=w803, y=w804) -> (x*y=w802:dbl)
                n310 = Add(x=w806, y=w800) -> (x+y=w805:dbl)
                n311 = Add(x=w802, y=w800) -> (x+y=w801:dbl)
              }
            }
            n312 = In Range and Coerce(upper limit=w774, x=w779, lower limit=w775) -> (coerced(x)=w778:dbl)  [unwired: 1 out]
            n313 = In Range and Coerce(upper limit=w774, x=w777, lower limit=w775) -> (coerced(x)=w776:dbl)  [unwired: 1 out]
            n314 = for {
              tunnel: w797 -> [w817] mode=indexing
              tunnel: w786 -> [w822]
              tunnel: w780 -> [w821]
              tunnel: w776 -> [w819]
              tunnel: w778 -> [w818]
              shift-right: [w815] -> w773
              shift-left: w782 -> [w816]
              shift-right: [w812] -> w781
              shift-left: w782 -> [w813]
              i -> [w823]
              stop <- w809 stop-if-true
              n315 = Multiply(x=w822, y=w823) -> (x*y=w820:dbl)
              n316 = Add(x=w821, y=w820) -> (x+y=w814:dbl)
              n317 = In Range and Coerce(upper limit=w819, x=w814, lower limit=w818) -> (In Range?=w810:bool)  [unwired: 1 out]
              n318 = case shown="True" w810 {
                tunnel: w817 -> [_ w831]
                tunnel: w816 -> [w825 w830]
                tunnel: [w825 w829] -> w815
                tunnel: w814 -> [_ w828]
                tunnel: w813 -> [w824 w827]
                tunnel: [w824 w826] -> w812
                frame False {
                }
                frame True {
                  n319 = Build Array (concatenate)(w827, w828) -> (w826:dbl[])
                  n320 = Build Array (concatenate)(w830, w831) -> (w829:dbl[])
                }
              }
              n321 = Array Size(array=w812) -> (size(s)=w811:i32)
              n322 = Greater Than 0?(x=w811) -> (x > 0?=w808:bool)
              n323 = Compound Arithmetic op=AND(invert w810, w808) -> (w809:bool)
            }
            n324 = Array Max & Min(array=w773) -> (max value=w767:dbl, min value=w766:dbl)  [unwired: 2 out]
            n325 = Array Size(array=w781) -> (size(s)=w796:i32)
            n326 = Absolute Value(x=w767) -> (abs(x)=w769:dbl)
            n327 = Absolute Value(x=w766) -> (abs(x)=w768:dbl)
            n328 = Decrement(x=w796) -> (x-1=w770:i32)
            n329 = Subtract(x=w769, y=w768) -> (x-y=w765:dbl)
            n330 = Equal To 0?(x=w770) -> (x = 0?=w771:bool)
            n331 = Subtract(x=w767, y=w772) -> (x-y=w793:dbl)
            n332 = Index Array(array=w781) -> (element=w795:dbl)  [unwired: 1 in]
            n333 = Index Array(array=w781, index=w770) -> (element=w794:dbl)
            n334 = Build Array(w767, w767) -> (w789:dbl[])
            n335 = Build Array(w793, w793) -> (w790:dbl[])
            n336 = Build Array(w795, w794) -> (w791:dbl[])
            n337 = Bundle(cluster=w792, "X"=w791, "Y"=w789) -> (w788:cluster{"X":dbl[], "Y":dbl[]})
            n338 = Bundle(cluster=w792, "X"=w791, "Y"=w790) -> (w787:cluster{"X":dbl[], "Y":dbl[]})
          }
        }
      }
      n339 = case shown="\"Insertion Loss\"..\"Return Loss\"" w407 {
        tunnel: [w472 w476] -> w410
        tunnel: w406 -> [w471 w475]
        frame Default {
          n340 = case shown="8" w471 {
            tunnel: [TRUE FALSE] -> w472
            frame 8 {
            }
            frame Default {
            }
          }
        }
        frame "Insertion Loss".."Return Loss" {
          n341 = case shown="8" w475 {
            tunnel: [FALSE TRUE] -> w476
            frame 8 {
            }
            frame Default {
            }
          }
        }
      }
      n342 = case shown="True" w410 {
        tunnel: w409 -> [w469 w470]
        tunnel: [w468 w470] -> w408
        frame True {
          n343 = Unbundle By Name(w469) -> ("Formatted Values"=w467:dbl[])
          n344 = Negate(x=w467) -> (-x=w466:dbl[])
          n345 = Bundle By Name(cluster=w469, "Formatted Values"=w466) -> (w468:T11)
        }
        frame False {
        }
      }
      n346 = Absolute Value(x=w404) -> (abs(x)=w405:dbl[])
      n347 = case shown="8" w406 {
        tunnel: w415 -> [w482 w492]
        tunnel: [w480 w492] -> w414
        tunnel: w413 -> [w481 w491]
        tunnel: [w479 w491] -> w412
        frame 8 {
          n348 = for {
            tunnel: w482 -> [w490] mode=indexing
            tunnel: [w489] -> w479 mode=indexing
            n349 = Unbundle By Name(w490) -> ("Y"=w488:dbl[])
            n350 = Negate(x=w488) -> (-x=w487:dbl[])
            n351 = Bundle By Name(cluster=w490, "Y"=w487) -> (w489:cluster{"X":dbl[], "Y":dbl[]})
          }
          n352 = for {
            tunnel: w481 -> [w486] mode=indexing
            tunnel: [w485] -> w480 mode=indexing
            n353 = Unbundle By Name(w486) -> ("Y"=w484:dbl[])
            n354 = Negate(x=w484) -> (-x=w483:dbl[])
            n355 = Bundle By Name(cluster=w486, "Y"=w483) -> (w485:cluster{"X":dbl[], "Y":dbl[]})
          }
        }
        frame Default {
        }
      }
      n356 = Array Max & Min(array=w405) -> (max value=w403:dbl)  [unwired: 3 out]
      n357 = case shown="Default" w425 {
        tunnel: w424 -> [_ w497]
        tunnel: [errorcluster {"status"=TRUE, "code"=-100098, "source"="Ripple limit can not be applied with the current settings.  Increase the number of points measured in order to apply the ripple limit."} ("error in (no error)") w497] -> w423
        frame 0 {
        }
        frame Default {
        }
      }
      n358 = call "SP Create Segmented Mask.vi"("Reset"=w455, "error in"=w423, "x0"=w452, "dx"=w451, "Specification Cluster"=w414) -> ("error out"=w453:errorcluster, "Limit"=w421:cluster{"x0":dbl, "dx":dbl, "Y":dbl[]})  [unwired: 3 out]
      n359 = call "SP Create Segmented Mask.vi"("Reset"=w455, "error in"=w423, "x0"=w452, "dx"=w451, "Specification Cluster"=w412) -> ("error out"=w454:errorcluster, "Limit"=w422:cluster{"x0":dbl, "dx":dbl, "Y":dbl[]})  [unwired: 3 out]
      n360 = Unbundle(w421) -> ("x0"=w435:dbl, "dx"=w434:dbl, "Y"=w433:dbl[])
      n361 = Unbundle(w422) -> ("x0"=w428:dbl, "dx"=w429:dbl, "Y"=w430:dbl[])
      n362 = Merge Errors(w453, w454) -> (w457:errorcluster)
      n363 = call "SP Format Value to Fundamental (array).vi"("Sxx Display Format"=w407, "Display Values"=w433) -> ("Stored Values"=w432:dbl[])  [unwired: 5 out]
      n364 = call "SP Format Value to Fundamental (array).vi"("Sxx Display Format"=w407, "Display Values"=w430) -> ("Stored Values"=w431:dbl[])  [unwired: 5 out]
      n365 = Build Array(w422) -> (w444:cluster{"x0":dbl, "dx":dbl, "Y":dbl[]}[])
      n366 = Build Array(w421) -> (w443:cluster{"x0":dbl, "dx":dbl, "Y":dbl[]}[])
      n367 = Bundle("x0"=w435, "dx"=w434, "Stored Values"=w432) -> (w417:T21)  [unwired: 1 out]
      n368 = Bundle("x0"=w428, "dx"=w429, "Stored Values"=w431) -> (w416:T21)  [unwired: 1 out]
      n369 = call "SP Convert Waveform to X-Y.vi"("Waveform"=w408) -> ("X-Y"=w441:cluster{"X":dbl[], "Y":dbl[]})
      n370 = Bundle(w417, w416) -> (w427:T22)  [unwired: 1 out]
      n371 = call "SP Perform Limit Testing.vi"("Generate Plot Output? (f)"=w426, "error in (no error)"=w457, "LLimits"=w444, "ULimits"=w443, "Data"=w408) -> ("error out"=w458:errorcluster, "Lower Pass?"=w438:bool, "Upper Pass?"=w439:bool, "Failures"=w440:cluster{"x values":dbl[], "y values":dbl[]}[])  [unwired: 2 in, 1 out]
      n372 = And(x=w439, y=w438) -> (x .and. y?=w436:bool)
      n373 = Build Array (concatenate)(w441, w440, w414, w412) -> (w442:cluster{"X":dbl[], "Y":dbl[]}[])
      n374 = Bundle("Upper Pass?"=w439, "Lower Pass?"=w438) -> (w437:cluster{"Upper Pass?":bool, "Lower Pass?":bool})  [unwired: 1 out]
    }
  }
  "Limits Pass/Fail" <- w9
  "Upper and Lower Limits" <- w8
  "Plot Output" <- w6
  "error out" <- w17
  "Upper Limits" <- w13
  "Lower Limits" <- w14
  "Failures" <- w12
  n375 = Bundle By Name(cluster="Limit Results In", "Ripple Pass?.Pass?"=w4, "Ripple Pass?.Ripple"=w3, "Ripple Pass?.Limit"=w2, "Ripple Pass?.Format"=w1) -> (→"Limit Results Out":T2)
